vi "Test AO Configuration.vi"(8 "error in (no error)":errorcluster, 11 "Instrument.Lockin in":refnum<class "Instrument.Lockin.lvclass">) -> (0 "error out":errorcluster, 3 "Instrument.Lockin out":refnum<class "Instrument.Lockin.lvclass">)   [LabVIEW 2016]
uses:
  src/Instrument.Lockin/Instrument.Lockin.lvclass
  src/LockinDAQ/Typedefs/AO-cluster.ctl
  src/LockinDAQ/Typedefs/AO_Amp-array.ctl
  src/LockinDAQ/Typedefs/AO_DC-array.ctl
  src/LockinDAQ/Typedefs/AO_f-array.ctl
  src/LockinDAQ/Typedefs/AO_phi-array.ctl
  src/LockinDAQ/Typedefs/Function-array.ctl
  src/LockinDAQ/Typedefs/Function-enum.ctl
  <vilib>/addons/_JKI Toolkits/Caraya/classes/Assert/Assert Equal Value and Type_Variant.vi
  <userlib>/_OpenG.lib/numeric/numeric.llb/Random Number Within Range - I32__ogtk.vi
  <userlib>/_OpenG.lib/numeric/numeric.llb/Random Number Within Range - DBL__ogtk.vi
  <vilib>/addons/_JKI Toolkits/Caraya/classes/Assert/Assert Almost Equal_Float.vi
  <vilib>/addons/_JKI Toolkits/Caraya/classes/Assert/Assert Equal Value_Variant.vi
  src/LockinDAQ/LockinDAQ.lvclass
  <vilib>/addons/_JKI Toolkits/Caraya/classes/Test/Test.lvclass
  <vilib>/addons/_JKI Toolkits/Caraya/classes/Assert/Assert.lvclass
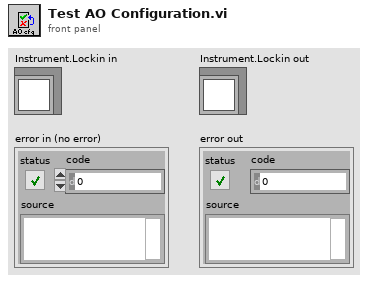
[diagram p1: front panel]
types:
  T1 = typedef "LockinDAQ.lvclass/AO-cluster.ctl" = cluster{"AO Amp (V)":T2, "AO DC (V)":T3, "AO f (Hz)":T4, "AO Phase (°)":T5, "Function":T6, "I+":bool[], "Sweeping":bool[]}
  T2 = typedef "LockinDAQ.lvclass/AO_Amp-array.ctl" = dbl[]
  T3 = typedef "LockinDAQ.lvclass/AO_DC-array.ctl" = dbl[]
  T4 = typedef "LockinDAQ.lvclass/AO_f-array.ctl" = dbl[]
  T5 = typedef "LockinDAQ.lvclass/AO_phi-array.ctl" = dbl[]
  T6 = typedef "LockinDAQ.lvclass/Function-array.ctl" = T7[]
  T7 = typedef "LockinDAQ.lvclass/Function-enum.ctl" = enum16{"Sine", "Triangle", "Square", "Sawtooth"}
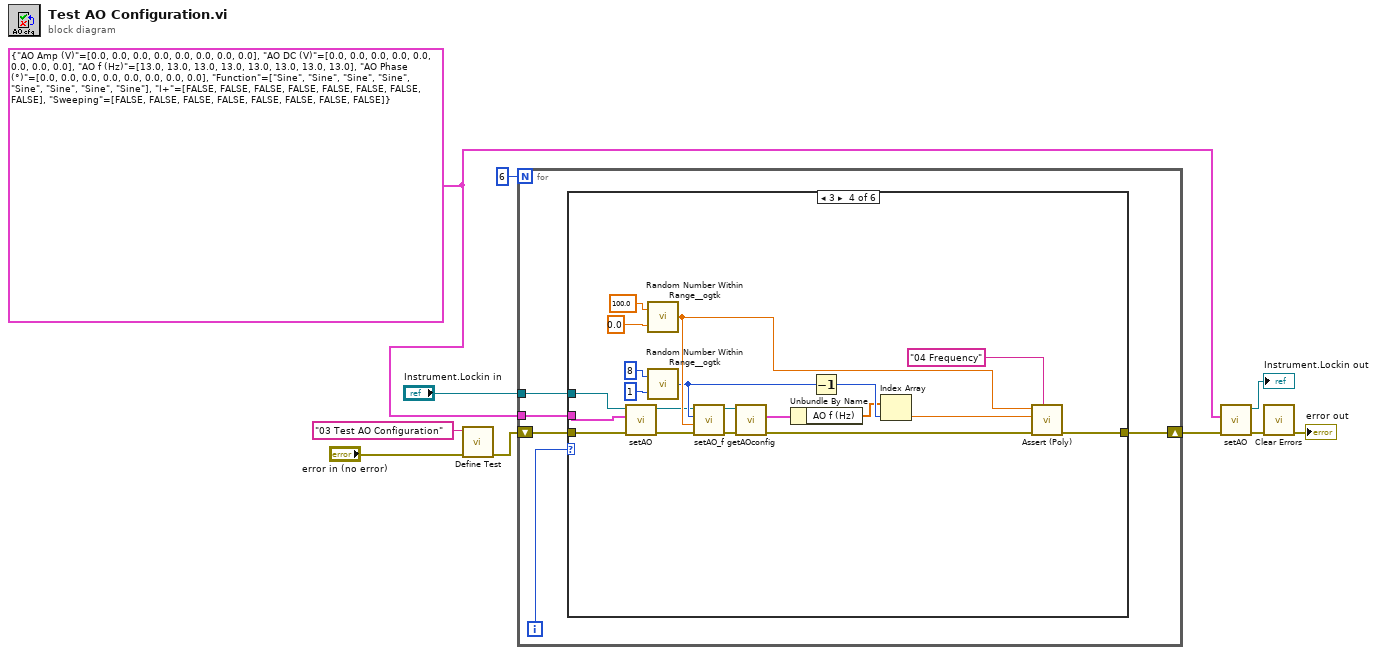
[diagram p0: block diagram]
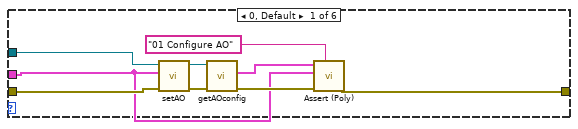
[diagram p2: hidden frame]
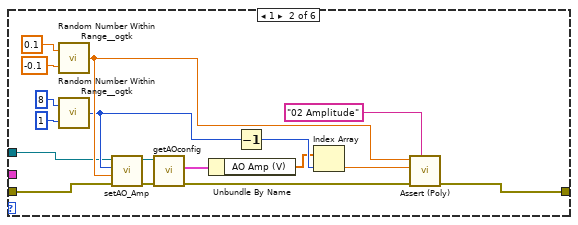
[diagram p3: hidden frame]
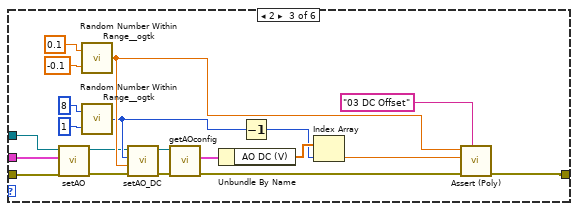
[diagram p4: hidden frame]
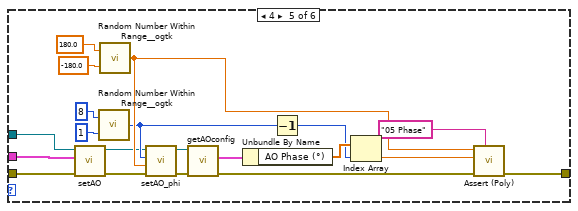
[diagram p5: hidden frame]
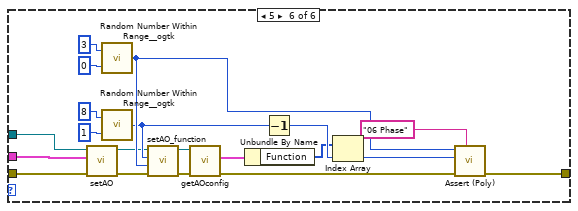
[diagram p6: hidden frame]
diagram:
  w5 = T1 {"AO Amp (V)"=[0.0, 0.0, 0.0, 0.0, 0.0, 0.0, 0.0, 0.0], "AO DC (V)"=[0.0, 0.0, 0.0, 0.0, 0.0, 0.0, 0.0, 0.0], "AO f (Hz)"=[13.0, 13.0, 13.0, 13.0, 13.0, 13.0, 13.0, 13.0], "AO Phase (°)"=[0.0, 0.0, 0.0, 0.0, 0.0, 0.0, 0.0, 0.0], "Function"=[enum."Sine", enum."Sine", enum."Sine", enum."Sine", enum."Sine", enum."Sine", enum."Sine", enum."Sine"], "I+"=[FALSE, FALSE, FALSE, FALSE, FALSE, FALSE, FALSE, FALSE], "Sweeping"=[FALSE, FALSE, FALSE, FALSE, FALSE, FALSE, FALSE, FALSE]} ("Channels: AO")
  n1 = call <vilib>:"Define Test.vi"("error in (no error)"="error in (no error)", "Label (VI Title)"="03 Test AO Configuration") -> ("error out"=w4:errorcluster)  [unwired: 9 in]
  n2 = for {
    N: 6 -> [_]
    tunnel: "Instrument.Lockin in" -> [w13]
    tunnel: w5 -> [w12]
    shift-right: [w11] -> w6
    shift-left: w4 -> [w14]
    i -> [w15]
    n3 = case shown="3" w15 {
      tunnel: w13 -> [w20 w26 w44 w64 w84 w104]
      tunnel: w14 -> [w18 w28 w45 w66 w83 w103]
      tunnel: w12 -> [w16 _ w43 w65 w85 w105]
      tunnel: [w19 w25 w42 w63 w82 w102] -> w11
      frame 0, Default {
        n4 = call "setAO.vi"("error in (no error)"=w18, "Channels: AO"=w16, "Instrument.Lockin in"=w20) -> ("error out"=w21:errorcluster, "Instrument.Lockin out"=w22:refnum<class "Instrument.Lockin.lvclass">)  [unwired: 7 in]
        n5 = call "getAOconfig.vi"("error in (no error)"=w21, "Instrument.Lockin in"=w22) -> ("error out"=w24:errorcluster, "AOconfig"=w23:T1)  [unwired: 7 in, 1 out]
        n6 = call-poly <vilib>:"Assert (Poly).vi"("Label"="01 Configure AO", "error in (no error)"=w24, "Y"=w16, "X"=w23) -> ("error out"=w19:errorcluster)  [unwired: 7 in]
      }
      frame 1 {
        n7 = call-poly <userlib>:"Random Number Within Range__ogtk.vi"("High"=0.1, "Low"=-0.1) -> ("Random Number"=w39:dbl)  [unwired: 3 in]
        n8 = call-poly <userlib>:"Random Number Within Range__ogtk.vi"("High"=8, "Low"=1) -> ("Random Number"=w35:i32)  [unwired: 3 in]
        n9 = call "setAO_Amp.vi"("error in (no error)"=w28, "Amplitude (V)"=w39, "AO Channel"=w35, "Instrument.Lockin in"=w26) -> ("error out"=w29:errorcluster, "Instrument.Lockin out"=w30:refnum<class "Instrument.Lockin.lvclass">)  [unwired: 6 in]
        n10 = call "getAOconfig.vi"("error in (no error)"=w29, "Instrument.Lockin in"=w30) -> ("error out"=w41:errorcluster, "AOconfig"=w31:T1)  [unwired: 7 in, 1 out]
        n11 = Unbundle By Name(w31) -> ("AO Amp (V)"=w32:T2)
        n12 = Decrement(x=w35) -> (x-1=w33:i32)
        n13 = Index Array(array=w32, index=w33) -> (element=w40:dbl)
        n14 = call-poly <vilib>:"Assert (Poly).vi"("Label"="02 Amplitude", "error in (no error)"=w41, "Y"=w40, "X"=w39) -> ("error out"=w25:errorcluster)  [unwired: 7 in]
      }
      frame 2 {
        n15 = call "setAO.vi"("error in (no error)"=w45, "Channels: AO"=w43, "Instrument.Lockin in"=w44) -> ("error out"=w53:errorcluster, "Instrument.Lockin out"=w52:refnum<class "Instrument.Lockin.lvclass">)  [unwired: 7 in]
        n16 = call-poly <userlib>:"Random Number Within Range__ogtk.vi"("High"=0.1, "Low"=-0.1) -> ("Random Number"=w61:dbl)  [unwired: 3 in]
        n17 = call-poly <userlib>:"Random Number Within Range__ogtk.vi"("High"=8, "Low"=1) -> ("Random Number"=w58:i32)  [unwired: 3 in]
        n18 = call "setAO_DC.vi"("error in (no error)"=w53, "DC (V)"=w61, "AO Channel"=w58, "Instrument.Lockin in"=w52) -> ("error out"=w46:errorcluster, "Instrument.Lockin out"=w47:refnum<class "Instrument.Lockin.lvclass">)  [unwired: 6 in]
        n19 = call "getAOconfig.vi"("error in (no error)"=w46, "Instrument.Lockin in"=w47) -> ("error out"=w60:errorcluster, "AOconfig"=w59:T1)  [unwired: 7 in, 1 out]
        n20 = Unbundle By Name(w59) -> ("AO DC (V)"=w57:T3)
        n21 = Decrement(x=w58) -> (x-1=w56:i32)
        n22 = Index Array(array=w57, index=w56) -> (element=w55:dbl)
        n23 = call-poly <vilib>:"Assert (Poly).vi"("Label"="03 DC Offset", "error in (no error)"=w60, "Y"=w55, "X"=w61) -> ("error out"=w42:errorcluster)  [unwired: 7 in]
      }
      frame 3 {
        n24 = call "setAO.vi"("error in (no error)"=w66, "Channels: AO"=w65, "Instrument.Lockin in"=w64) -> ("error out"=w70:errorcluster, "Instrument.Lockin out"=w69:refnum<class "Instrument.Lockin.lvclass">)  [unwired: 7 in]
        n25 = call-poly <userlib>:"Random Number Within Range__ogtk.vi"("High"=100.0, "Low"=0.0) -> ("Random Number"=w79:dbl)  [unwired: 3 in]
        n26 = call-poly <userlib>:"Random Number Within Range__ogtk.vi"("High"=8, "Low"=1) -> ("Random Number"=w78:i32)  [unwired: 3 in]
        n27 = call "setAO_f.vi"("error in (no error)"=w70, "Frequency (Hz)"=w79, "AO Channel"=w78, "Instrument.Lockin in"=w69) -> ("error out"=w67:errorcluster, "Instrument.Lockin out"=w68:refnum<class "Instrument.Lockin.lvclass">)  [unwired: 6 in]
        n28 = call "getAOconfig.vi"("error in (no error)"=w67, "Instrument.Lockin in"=w68) -> ("error out"=w81:errorcluster, "AOconfig"=w80:T1)  [unwired: 7 in, 1 out]
        n29 = Unbundle By Name(w80) -> ("AO f (Hz)"=w71:T4)
        n30 = Decrement(x=w78) -> (x-1=w72:i32)
        n31 = Index Array(array=w71, index=w72) -> (element=w73:dbl)
        n32 = call-poly <vilib>:"Assert (Poly).vi"("Label"="04 Frequency", "error in (no error)"=w81, "Y"=w73, "X"=w79) -> ("error out"=w63:errorcluster)  [unwired: 7 in]
      }
      frame 4 {
        n33 = call "setAO.vi"("error in (no error)"=w83, "Channels: AO"=w85, "Instrument.Lockin in"=w84) -> ("error out"=w101:errorcluster, "Instrument.Lockin out"=w88:refnum<class "Instrument.Lockin.lvclass">)  [unwired: 7 in]
        n34 = call-poly <userlib>:"Random Number Within Range__ogtk.vi"("High"=8, "Low"=1) -> ("Random Number"=w98:i32)  [unwired: 3 in]
        n35 = call-poly <userlib>:"Random Number Within Range__ogtk.vi"("High"=180.0, "Low"=-180.0) -> ("Random Number"=w99:dbl)  [unwired: 3 in]
        n36 = call "setAO_phi.vi"("error in (no error)"=w101, "Phase (°)"=w99, "AO Channel"=w98, "Instrument.Lockin in"=w88) -> ("error out"=w86:errorcluster, "Instrument.Lockin out"=w87:refnum<class "Instrument.Lockin.lvclass">)  [unwired: 6 in]
        n37 = call "getAOconfig.vi"("error in (no error)"=w86, "Instrument.Lockin in"=w87) -> ("error out"=w100:errorcluster, "AOconfig"=w97:T1)  [unwired: 7 in, 1 out]
        n38 = Unbundle By Name(w97) -> ("AO Phase (°)"=w96:T5)
        n39 = Decrement(x=w98) -> (x-1=w95:i32)
        n40 = Index Array(array=w96, index=w95) -> (element=w94:dbl)
        n41 = call-poly <vilib>:"Assert (Poly).vi"("Label"="05 Phase", "error in (no error)"=w100, "Y"=w94, "X"=w99) -> ("error out"=w82:errorcluster)  [unwired: 7 in]
      }
      frame 5 {
        n42 = call "setAO.vi"("error in (no error)"=w103, "Channels: AO"=w105, "Instrument.Lockin in"=w104) -> ("error out"=w109:errorcluster, "Instrument.Lockin out"=w108:refnum<class "Instrument.Lockin.lvclass">)  [unwired: 7 in]
        n43 = call-poly <userlib>:"Random Number Within Range__ogtk.vi"("High"=3, "Low"=0) -> ("Random Number"=w120:i32)  [unwired: 3 in]
        n44 = call-poly <userlib>:"Random Number Within Range__ogtk.vi"("High"=8, "Low"=1) -> ("Random Number"=w117:i32)  [unwired: 3 in]
        n45 = call "setAO_function.vi"("error in (no error)"=w109, "Function"=w120, "AO Channel"=w117, "Instrument.Lockin in"=w108) -> ("error out"=w106:errorcluster, "Instrument.Lockin out"=w107:refnum<class "Instrument.Lockin.lvclass">)  [unwired: 6 in]
        n46 = call "getAOconfig.vi"("error in (no error)"=w106, "Instrument.Lockin in"=w107) -> ("error out"=w121:errorcluster, "AOconfig"=w116:T1)  [unwired: 7 in, 1 out]
        n47 = Unbundle By Name(w116) -> ("Function"=w110:T6)
        n48 = Decrement(x=w117) -> (x-1=w111:i32)
        n49 = Index Array(array=w110, index=w111) -> (element=w112:T7)
        n50 = call-poly <vilib>:"Assert (Poly).vi"("Label"="06 Phase", "error in (no error)"=w121, "Y"=w112, "X"=w120) -> ("error out"=w102:errorcluster)  [unwired: 7 in]
      }
    }
  }
  n51 = call "setAO.vi"("error in (no error)"=w6, "Channels: AO"=w5) -> ("error out"=w9:errorcluster, "Instrument.Lockin out"=→"Instrument.Lockin out":refnum<class "Instrument.Lockin.lvclass">)  [unwired: 8 in]
  n52 = call <vilib>:"Clear Errors.vi"("error in (no error)"=w9) -> ("error out"=→"error out":errorcluster)  [unwired: 5 in, 1 out]
